vi "10-Tap 8-bit Camera without DRAM (FPGA-SIM)WithoutSCTLAccum.vi"() -> ()   [LabVIEW 2013]
doc: "This is the FPGA VI for the 10-Tap 8-Bit Camera with DRAM example. This example demonstrates how to acquire images from a 10-tap, 8-bit, extended configuration, Camera Link camera and transfer the images to the host. This example supports area scan and line scan cameras for both continuous and finite acquisitions.\n\nThis example also demonstrates the use of DRAM as a frame buffer for very high speed acquisitions. Data packing and flow-control are also employed to maximize use of the available DRAM and FIFOs in terms of both memory space and performance.\n\nAdditionally, the example demonstrates the serial server, which allows third-party camera configuration utilities to communicate with the camera using the Camera Link serial interface while this VI is running."
uses:
  Common/CL Signal Mapping.ctl
  Common/CL Configuration.ctl
  FPGA/Sector/Accumulate/Sector Parameter Cluster.ctl
  <vilib>/Platform/TimedLoop/XDataNode/timing_clust.ctl
  <vilib>/Platform/TimedLoop/XDataNode/nitl_modes.ctl
  <vilib>/Platform/TimedLoop/XDataNode/wakeup.ctl
  <vilib>/rvi/Emulation/niFpgaSctlEmulationGetInTimedLoop.vi
  <vilib>/rvi/Emulation/niFpgaEmulationReportErrorSimple.vi
  <vilib>/rvi/Emulation/niFpgaGetClockAttributes.vi
  <vilib>/rvi/Emulation/niFpgaCriticalErrorInLSC.vi
  <vilib>/rvi/FIFO/Fifo_Resource/nirvififoEmulationGetNumberOfElementsToWriteFpgaImpl.vi
  <vilib>/rvi/DataTransferAndStorage/Container/Common/niFpgaContainerGetUniqueNameForEmu.vi
  <vilib>/rvi/interface/RandomDataEmulation/nirviRandomDataFPGAFIFO.vi
  <vilib>/rvi/interface/RandomDataEmulation/niFpgaRandomDataHandleErrors.vi
  <vilib>/rvi/FIFO/Fifo_Resource/nirvififoEmulationWriteFpgaImpl.vi
  <vilib>/rvi/FIFO/Fifo_Resource/nirvififoEmulationReadFpgaImpl.vi
  <vilib>/rvi/FIFO/Fifo_Resource/nirvififoEmulationGetNumberOfElementsToReadFpgaImpl.vi
  <vilib>/rvi/Emulation/niFpgaProcessEmulError.vi
  FPGA/Globals/Pixel Location Global.vi
  FPGA/Globals/Sector Parameter Global.vi
  FPGA/Globals/Accumulated Sector Intensity.vi
  <vilib>/Platform/TimedLoop/XDataNode/XDataNode.xnode
  <vilib>/rvi/DataTransferAndStorage/Container/XNode/niFpgaContainer.xnode
  <vilib>/rvi/FIFO/Fifo_Resource/nirvififoEmulationGetNumberOfElementsToWrite.vi
  <vilib>/rvi/interface/RandomDataEmulation/nirviRandomDataFpgaReadWriteTemplate.vi
  <vilib>/rvi/FIFO/Fifo_Resource/nirvififoEmulationWrite.vi
  <vilib>/rvi/FIFO/Fifo_Resource/nirvififoEmulationRead.vi
  <vilib>/rvi/FIFO/Fifo_Resource/nirvififoEmulationGetNumberOfElementsToRead.vi
  <vilib>/Platform/TimedLoop/XDataNode/XDNodeRunTimeDep.lvlib
  FPGA/Globals/Wing Square Wave Frequency Global.vi
panel:
  out "Number of Elements to Write Sector Grouping FIFO":u32
  out "Accumulate Ticks":u32
  out "Analysis Ticks":u32
  out "Target Sim TO":bool
  out "Cam Data Timeout":bool
  out "Sector FIFO Timeout":bool
  out "Host DMA Timeout":bool
  out "Number of Elements to Read Cam Data":u32
  out "Number of Elements to Write Host DMA":u32
  in  "Words per image":u32=1000
  in  "Y Resolution":u16=1000
  in  "X Resolution":u16=1000
  in  "[Average BG Intensity]":u8[](array[numeric])=[0, 0, 0, 0, 0, 0, 0, 0, 0, 0, 0, 0, 0, 0, 0, 0, 0, 0, 0, 0, 0, 0, 0, 0, 0, 0, 0, 0, 0, 0, 0, 0]
  in  "Sector Threshold":u8
  in  "# of Frames to Average":u8=1
  in  "Sector Parameters Right":T1={"Start Angle"=0.0, "End Angle"=0.4708251953125, "Inner Radius"=309, "Outter Radius"=405, "Hinge X"=685, "Hinge Y"=527, "NumWingSectors"=8}
  in  "Sector Parameters Left":T1={"Start Angle"=0.65740966796875, "End Angle"=0.99468994140625, "Inner Radius"=309, "Outter Radius"=405, "Hinge X"=464, "Hinge Y"=534, "NumWingSectors"=8}
  in  "CL Config.Configuration":T2=enum."Full"
  in  "CL Config.Signal Mapping":T3=enum."Basler 10-tap"
  in  "CL Config.Line Scan":bool
  in  "CL Config.DVAL Active High":bool=TRUE
  in  "CL Config.LVAL Active High":bool=TRUE
  in  "CL Config.FVAL Active High":bool=TRUE
  in  "CL Config.Spare Active High":bool=TRUE
  in  "Acq Control.Line Scan Height":u32
  in  "Acq Control.Frames To Acq":u32
  in  "Acq Control.Acquire":bool
  in  "Acq Control.Cancel Acq":bool
  in  "Acq Control.Ignore DVAL":bool
  in  "Acq Control.Initialize":bool
  out "Acq Status.Acq In Progress":bool
  out "Acq Status.Clocks Per Line":u32
  out "Acq Status.Frames Acq'd":u32
  out "Acq Status.Lines Per Frame":u32
  out "Acq Status.DMA Write Timeout":bool
  out "Acq Status.Initialized":bool
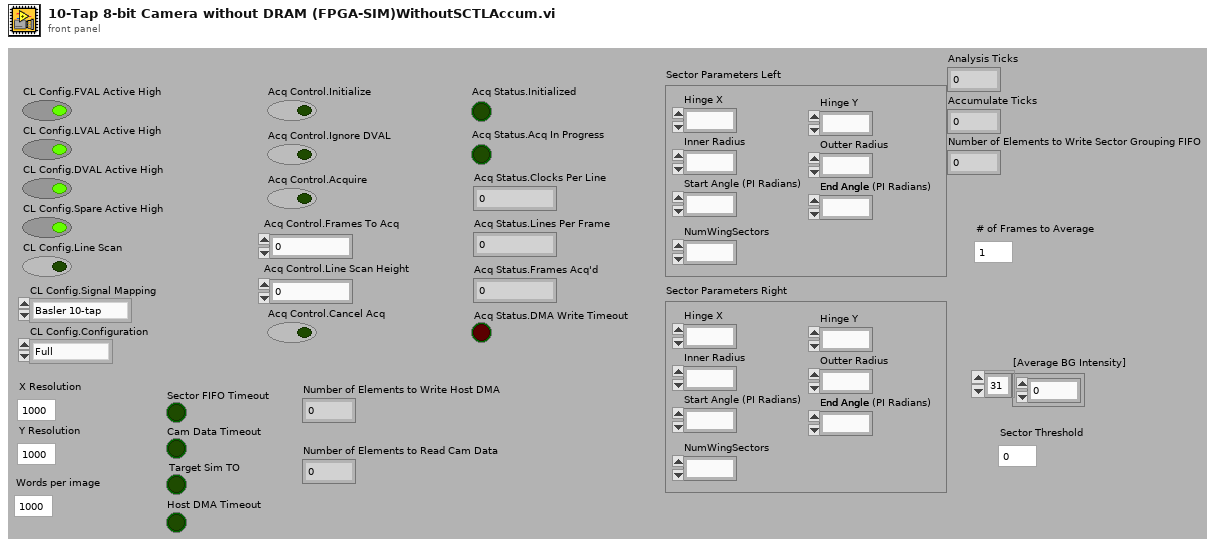
[diagram p1: front panel]
types:
  T1 = typedef "Sector Parameter Cluster.ctl" = cluster{"Start Angle":fxp<+/-,17,2>, "End Angle":fxp<+,17,3>, "Inner Radius":u16, "Outter Radius":u16, "Hinge X":u16, "Hinge Y":u16, "NumWingSectors":u8}
  T2 = typedef "CL Configuration.ctl" = enum8{"Base", "Medium", "Full"}
  T3 = typedef "CL Signal Mapping.ctl" = enum8{"Standard", "Basler 10-tap", "Vosskühler 10-tap"}
  T4 = typedef "XDNodeRunTimeDep.lvlib/timing_clust.ctl" = cluster{"Expected End [f-1]":u64, "Actual End [f-1]":u64, "Finished Late? [f-1]":bool, "Expected End [i-1]":u64, "Actual End [i-1]":u64, "Finished Late? [i-1]":bool, "Expected Start [i]":u64, "Actual Start [i]":u64, "Expected Start [f]":u64, "Actual Start [f]":u64, "Source Name":string, "Structure Name":string, "Period":i64, "Deadline":i64, "Offset":i64, "Start":i64, "Priority":i32, "Timeout":i32, "Mode":T5, "Wakeup Reason":T6, "Error":errorcluster, "Source Type":string, "Secondary Source Type":string, "Global End Time":u64, "Global Start Time":u64, "Frame Duration":u64, "Iteration Duration":u64, "Assigned CPU":i32, "I/O Scan Engine Mode":u32}
  T5 = typedef "XDNodeRunTimeDep.lvlib/nitl_modes.ctl" = enum32{"No Change", "Process missed periods, maintain original phase", "Discard missed periods, maintain original phase", "Process missed periods, ignore original phase", "Discard missed periods, ignore original phase"}
  T6 = typedef "XDNodeRunTimeDep.lvlib/wakeup.ctl" = enum32{"Normal", "Aborted", "Asynchronous wakeup", "Timing source error", "Timed loop error", "Timeout"}
  T7 = cluster{"Accumulated Intensity":u32, "Count":u16}[]
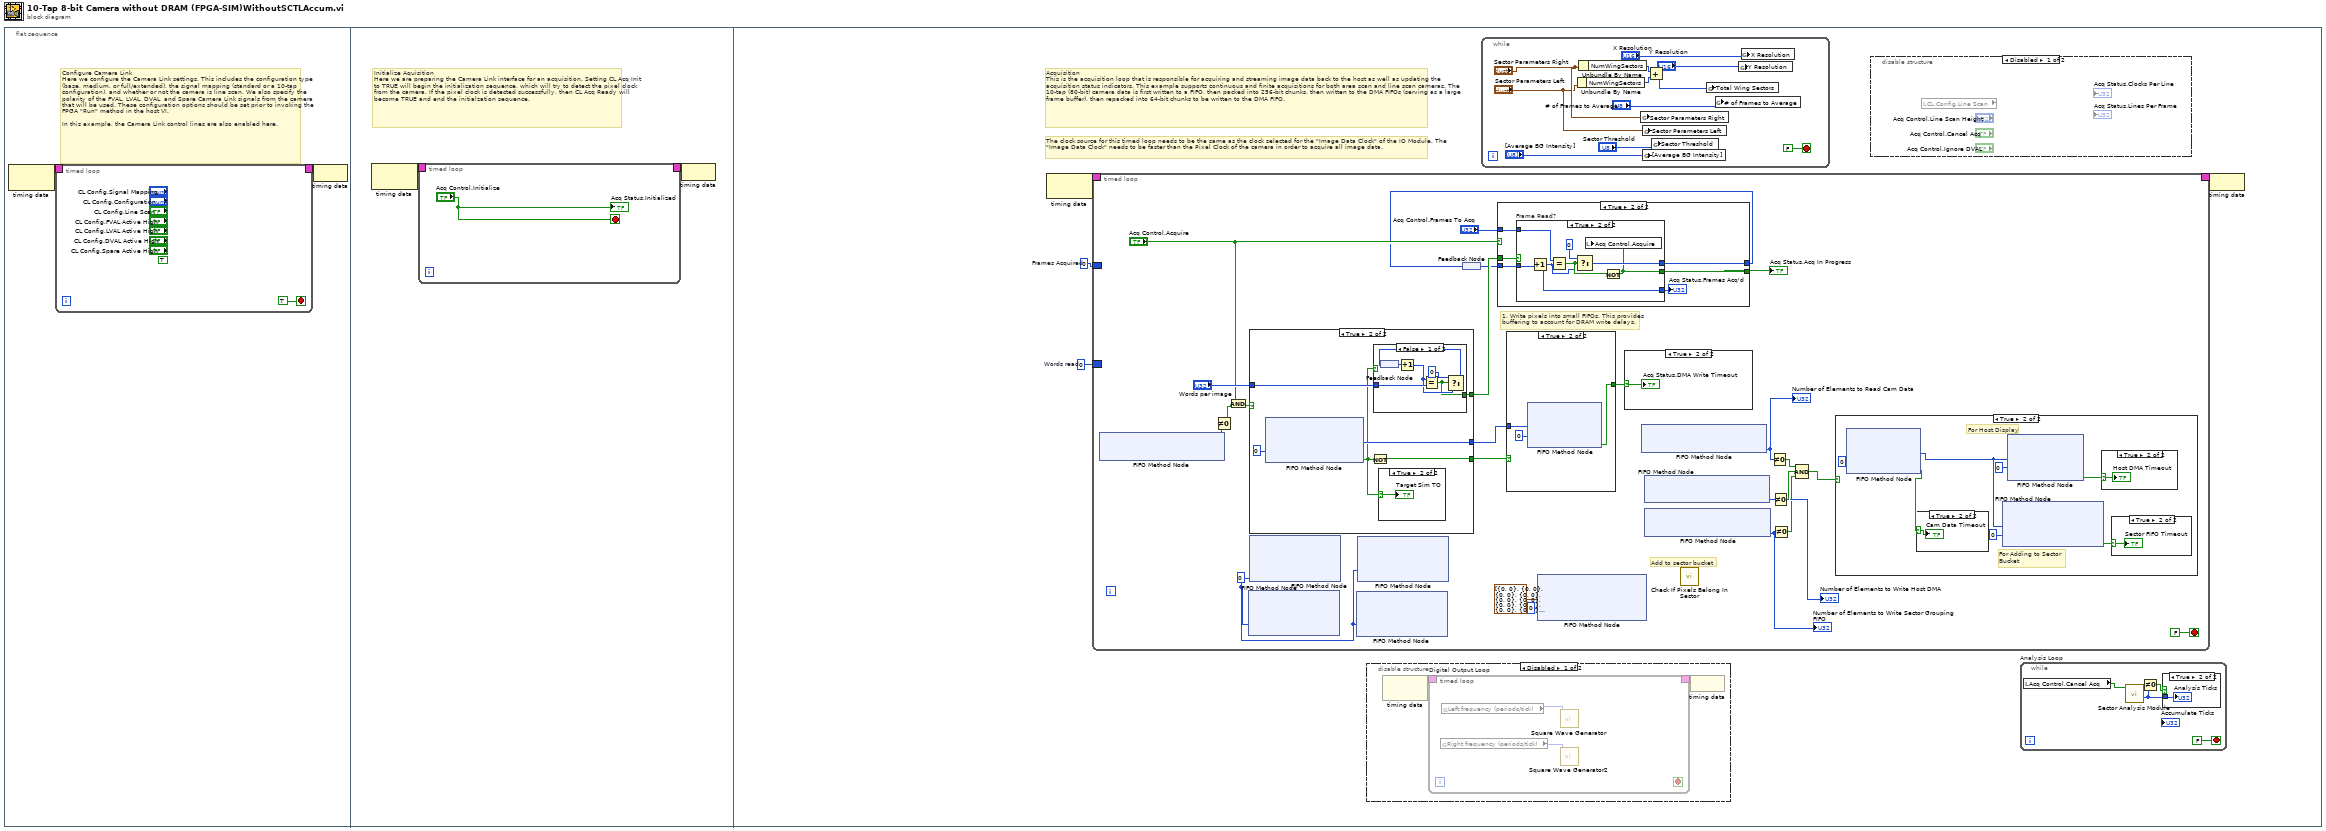
[diagram p0: block diagram]
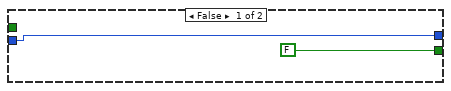
[diagram p6: hidden frame]
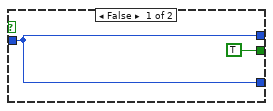
[diagram p7: hidden frame]
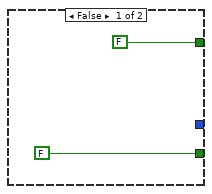
[diagram p8: hidden frame]
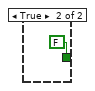
[diagram p10: hidden frame]
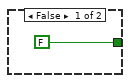
[diagram p15: hidden frame]
diagram:
  n1 = flat-sequence {
    frame #0 {
      # "Configure Camera Link\nHere we configure the Camera Link settings. This includes the configuration type (base, medium, or full/extended), the signal mapping (standard or a 10-tap configuration), and whether or not the camera is line scan. We also specify the polarity of the FVAL, LVAL, DVAL, and Spare Camera Link signals from the camera that will be used. These configuration options should be set prior to invoking the FPGA \"Run\" method in the host VI.\n\nIn this example, the Camera Link control lines are also enabled here."
      n2 = node-c288() -> (w2:T4)  [unwired: 1 in]
      n3 = timed-loop {
        timing: w2 -> [_]
        timing-out: [_] -> w1
        stop <- TRUE stop-if-true
        (unwired) TRUE ("IO Module\\CL Control Enable")
      }
      n4 = node-c288(w1) -> ()
    }
    frame #1 {
      # "Initialize Aquisition\nHere we are preparing the Camera Link interface for an acquisition. Setting CL Acq Init to TRUE will begin the initialization sequence, which will try to detect the pixel clock from the camera. If the pixel clock is detected successfully, then CL Acq Ready will become TRUE and end the initialzation sequence."
      n5 = node-c288() -> (w9:T4)  [unwired: 1 out]
      n6 = timed-loop {
        timing: w9 -> [_]
        timing-out: [_] -> w8
        stop <- "Acq Control.Initialize" stop-if-true
        "Acq Status.Initialized" <- "Acq Control.Initialize"
      }
      n7 = node-c288(w8) -> ()
    }
    frame #2 {
      w15 = u32 0  # Frames Acquired
      w16 = u32 0  # Words read
      # "The clock source for this timed loop needs to be the same as the clock selected for the \"Image Data Clock\" of the IO Module. The \"Image Data Clock\" needs to be faster than the Pixel Clock of the camera in order to acquire all image data."
      # "Acquisition\nThis is the acquisition loop that is responsible for acquiring and streaming image data back to the host as well as updating the acquisition status indicators. This example supports continuous and finite acquisitions for both area scan and line scan cameras. The 10-tap (80-bit) camera data is first written to a FIFO, then packed into 256-bit chunks, then written to the DMA FIFOs (serving as a large frame buffer), then repacked into 64-bit chunks to be written to the DMA FIFO."
      n8 = node-c288() -> (w18:T4)  [unwired: 1 in]
      n9 = timed-loop {
        timing: w18 -> [_]
        timing-out: [_] -> w17
        border: w16 -> [_]
        border: w15 -> [_]
        stop <- FALSE stop-if-true
        w37 = 0 ("Timeout")
        # "Add to sector bucket"
        # "1. Write pixels into small FIFOs. This provides\nbuffering to account for DRAM write delays."
        n10 = xnode ("FIFO Method Node")() -> ("Number of Elements to Write"=w49:u32)  [unwired: 1 in, 1 out]
        n11 = Not Equal To 0?(x=w49) -> (x != 0?=w48:bool)
        n12 = And(x="Acq Control.Acquire", y=w48) -> (x .and. y?=w56:bool)
        n13 = xnode ("FIFO Method Node")("Timeout"=w37) -> ()  [unwired: 1 in, 3 out]
        n14 = xnode ("FIFO Method Node")("Timeout"=w37) -> ()  [unwired: 1 in, 3 out]
        n15 = case shown="True" w56 {
          tunnel: [_ w86] -> w60
          tunnel: [FALSE w82] -> w58
          tunnel: "Words per image" -> [_ w84]
          tunnel: [FALSE w83] -> w45
          frame False {
          }
          frame True {
            n16 = xnode ("FIFO Method Node")("Timeout"=0) -> ("Element"=w86:u64, "Timed Out?"=w81:bool)  [unwired: 1 in, 1 out]
            n17 = Not(x=w81) -> (.not. x?=w82:bool)
            n18 = case shown="False" w81 {
              tunnel: w84 -> [w93 _]
              tunnel: [w88 FALSE] -> w83
              frame False {
                n19 = feedback #1() -> (w92:u32)
                n20 = Increment(x=w92) -> (x+1=w89:u32)
                n21 = Equal?(x=w89, y=w93) -> (x = y?=w88:bool)
                n22 = Select(t=u32 0 ("Acq Status.Frames Acq'd"), s=w88, f=w89) -> (s? t:f=w90:u32)
                n23 = feedback-in #1(w90) -> ()
              }
              frame True {
              }
            }
            n24 = case shown="True" w81 {
              selector: w81 -> [_ w87]
              frame False {
              }
              frame True {
                "Target Sim TO" <- w87
              }
            }
          }
        }
        n25 = xnode ("FIFO Method Node")("Timeout"=w37) -> ()  [unwired: 1 in, 3 out]
        n26 = xnode ("FIFO Method Node")("Timeout"=w37) -> ()  [unwired: 1 in, 3 out]
        n27 = feedback #2() -> (w44:u32)
        n28 = case shown="True" "Acq Control.Acquire" {
          tunnel: w45 -> [_ w69]
          tunnel: w44 -> [w63 w68]
          tunnel: "Acq Control.Frames To Acq" -> [_ w67]
          tunnel: [w63 w66] -> w42
          tunnel: [FALSE w65] -> w41
          frame False {
          }
          frame True {
            n29 = case "Frame Read?" shown="True" w69 {
              tunnel: w68 -> [w70 w78]
              tunnel: w67 -> [_ w77]
              tunnel: [w70 w75] -> w66
              tunnel: [TRUE w73] -> w65
              tunnel: [w70 w72] -> w64
              frame False {
              }
              frame True {
                n30 = Increment(x=w78) -> (x+1=w72:u32)
                n31 = Equal?(x=w77, y=w72) -> (x = y?=w74:bool)
                n32 = Select(t=u32 0 ("Frames Acquired"), s=w74, f=w72) -> (s? t:f=w75:u32)
                n33 = Not(x=w74) -> (.not. x?=w73:bool)
                n34 = local write "Acq Control.Acquire"(w73) -> ()
              }
            }
            "Acq Status.Frames Acq'd" <- w64
          }
        }
        "Acq Status.Acq In Progress" <- w41
        n35 = feedback-in #2(w42) -> ()
        n36 = case shown="True" w58 {
          tunnel: [FALSE ("Timed Out?") w107] -> w40
          tunnel: w60 -> [_ w108]
          frame False {
          }
          frame True {
            n37 = xnode ("FIFO Method Node")("Element"=w108, "Timeout"=0) -> ("Timed Out?"=w107:bool)  [unwired: 1 in, 1 out]
          }
        }
        n38 = xnode ("FIFO Method Node")("Element"=T7 [{"Accumulated Intensity"=0, "Count"=0}, {"Accumulated Intensity"=0, "Count"=0}, {"Accumulated Intensity"=0, "Count"=0}, {"Accumulated Intensity"=0, "Count"=0}, {"Accumulated Intensity"=0, "Count"=0}, {"Accumulated Intensity"=0, "Count"=0}, {"Accumulated Intensity"=0, "Count"=0}, {"Accumulated Intensity"=0, "Count"=0}, {"Accumulated Intensity"=0, "Count"=0}, {"Accumulated Intensity"=0, "Count"=0}, {"Accumulated Intensity"=0, "Count"=0}, {"Accumulated Intensity"=0, "Count"=0}, {"Accumulated Intensity"=0, "Count"=0}, {"Accumulated Intensity"=0, "Count"=0}, {"Accumulated Intensity"=0, "Count"=0}, {"Accumulated Intensity"=0, "Count"=0}, {"Accumulated Intensity"=0, "Count"=0}, {"Accumulated Intensity"=0, "Count"=0}, {"Accumulated Intensity"=0, "Count"=0}, {"Accumulated Intensity"=0, "Count"=0}, {"Accumulated Intensity"=0, "Count"=0}, {"Accumulated Intensity"=0, "Count"=0}, {"Accumulated Intensity"=0, "Count"=0}, {"Accumulated Intensity"=0, "Count"=0}, {"Accumulated Intensity"=0, "Count"=0}, {"Accumulated Intensity"=0, "Count"=0}, {"Accumulated Intensity"=0, "Count"=0}, {"Accumulated Intensity"=0, "Count"=0}, {"Accumulated Intensity"=0, "Count"=0}, {"Accumulated Intensity"=0, "Count"=0}, {"Accumulated Intensity"=0, "Count"=0}, {"Accumulated Intensity"=0, "Count"=0}], "Timeout"=0) -> ()  [unwired: 1 in, 2 out]
        n39 = case shown="True" w40 {
          selector: w40 -> [_ w61]
          frame False {
          }
          frame True {
            "Acq Status.DMA Write Timeout" <- w61
          }
        }
        n40 = xnode ("FIFO Method Node")() -> ("Number of Elements to Read"=w51:u32)  [unwired: 1 in, 1 out]
        "Number of Elements to Read Cam Data" <- w51
        n41 = xnode ("FIFO Method Node")() -> ("Number of Elements to Write"=w54:u32)  [unwired: 1 in, 1 out]
        "Number of Elements to Write Host DMA" <- w54
        n42 = xnode ("FIFO Method Node")() -> ("Number of Elements to Write"=w53:u32)  [unwired: 1 in, 1 out]
        "Number of Elements to Write Sector Grouping FIFO" <- w53
        n43 = call "Check If Pixels Belong In Sector.vi"() -> ()  [unwired: 11 in, 1 out]
        n44 = Not Equal To 0?(x=w51) -> (x != 0?=w50:bool)
        n45 = Not Equal To 0?(x=w54) -> (x != 0?=w55:bool)
        n46 = Not Equal To 0?(x=w53) -> (x != 0?=w52:bool)
        n47 = Compound Arithmetic op=AND(w50, w55, w52) -> (w57:bool)
        n48 = case shown="True" w57 {
          frame False {
          }
          frame True {
            # "For Adding to Sector \nBucket"
            # "For Host Display"
            n49 = xnode ("FIFO Method Node")("Timeout"=0) -> ("Element"=w99:u64, "Timed Out?"=w95:bool)  [unwired: 1 in, 1 out]
            n50 = case shown="True" w95 {
              selector: w95 -> [_ w102]
              frame False {
              }
              frame True {
                "Cam Data Timeout" <- w102
              }
            }
            n51 = xnode ("FIFO Method Node")("Element"=w99, "Timeout"=0) -> ("Timed Out?"=w97:bool)  [unwired: 1 in, 1 out]
            n52 = xnode ("FIFO Method Node")("Element"=w99, "Timeout"=0) -> ("Timed Out?"=w96:bool)  [unwired: 1 in, 1 out]
            n53 = case shown="True" w96 {
              selector: w96 -> [_ w103]
              frame False {
              }
              frame True {
                "Host DMA Timeout" <- w103
              }
            }
            n54 = case shown="True" w97 {
              selector: w97 -> [_ w104]
              frame False {
              }
              frame True {
                "Sector FIFO Timeout" <- w104
              }
            }
          }
        }
      }
      n55 = disable-structure shown="Disabled" {
        frame Disabled {
          n56 = node-c288() -> (w25:T4)  [unwired: 1 in]
          n57 = timed-loop "Digital Output Loop" {
            timing: w25 -> [_]
            timing-out: [_] -> w24
            stop <- _ stop-if-true
            n58 = global read "Wing Square Wave Frequency Global.vi" "Right frequency (periods/tick)"() -> (w26:fxp<+,32,0>)
            n59 = global read "Wing Square Wave Frequency Global.vi" "Left frequency (periods/tick)"() -> (w27:fxp<+,32,0>)
            n60 = call "Square Wave Generator"("frequency (periods/tick)"=w27) -> ()  [unwired: 14 in, 1 out]
            n61 = call "Square Wave Generator2"("frequency (periods/tick)"=w26) -> ()  [unwired: 14 in, 1 out]
          }
          n62 = node-c288(w24) -> ()
        }
        frame Enabled {
        }
      }
      n63 = while {
        stop <- FALSE stop-if-true
        n64 = Unbundle By Name("Sector Parameters Left") -> ("NumWingSectors"=w121:u8)
        n65 = Unbundle By Name("Sector Parameters Right") -> ("NumWingSectors"=w122:u8)
        n66 = global write "Sector Parameter Global.vi" "Sector Parameters Right"("Sector Parameters Right") -> ()
        n67 = global write "Sector Parameter Global.vi" "Sector Parameters Left"("Sector Parameters Left") -> ()
        n68 = global write "Sector Parameter Global.vi" "[Average BG Intensity]"("[Average BG Intensity]") -> ()
        n69 = Add(x=w122, y=w121) -> (x+y=w120:u8)
        n70 = global write "Sector Parameter Global.vi" "Sector Threshold"("Sector Threshold") -> ()
        n71 = global write "Accumulated Sector Intensity.vi" "Total Wing Sectors"(w120) -> ()
        n72 = global write "Pixel Location Global.vi" "# of Frames to Average"("# of Frames to Average") -> ()
        n73 = global write "Pixel Location Global.vi" "Y Resolution"("Y Resolution") -> ()
        n74 = global write "Pixel Location Global.vi" "X Resolution"("X Resolution") -> ()
      }
      n75 = disable-structure shown="Disabled" {
        frame Disabled {
          n76 = local read "CL Config.Line Scan"() -> (w21:bool)
        }
        frame Enabled {
        }
      }
      n77 = while "Analysis Loop" {
        stop <- FALSE stop-if-true
        n78 = local read "Acq Control.Cancel Acq"() -> (w34:bool)
        n79 = call "Sector Analysis Module.vi"("Canceled?"=w34) -> ("Analysis Ticks"=w33:u32)  [unwired: 9 in, 1 out]
        n80 = Not Equal To 0?(x=w33) -> (x != 0?=w32:bool)
        n81 = case shown="True" w32 {
          tunnel: w33 -> [_ w36]
          frame False {
          }
          frame True {
            "Analysis Ticks" <- w36
          }
        }
      }
      n82 = node-c288(w17) -> ()
    }
  }
